vi "Substitute Actor.vi"(10 "Substitute Actor in":refnum<class "Actor.lvclass">, 11 "Current State Machine Actor":refnum<class "State Machine Actor.lvclass">) -> (0 "error out":errorcluster, 2 "Substitute Actor out":refnum<class "Actor.lvclass">)   [LabVIEW 2024]
doc: "(<B>Filename</B>: Actor Framework.lvlib:Actor.lvclass:Substitute Actor.vi)\n\nThis method copies information from the <b>Current Actor</b> to the <b>Substitute Actor</b>, including the to-self and the to-caller queue references. The purpose of this function is to allow an actor to define a method that replaces itself with another actor, useful for implementing a State Pattern Actor. Child classes should override this method to copy any additional fields that they need from the current to the substitute.\n\nThis method may return error code 678010: Illegal substitution. Overrides of this method may choose to return this error if the new actor is not one that is an appropriate substitute for the current actor, for whatever standards of \"appropriate\" are chosen for the current actor. If returning an error, override VIs should return the unmodified <b>Current Actor</b> as <b>Substitute Actor out</b>."
uses:
  State Machine Actor.lvclass/State Machine Actor.ctl
  State Machine Actor.lvclass
  C:/Users/uspoaotto/OneDrive - Oregon Tool/Desktop/working copies/stateMachineActor/src/_State Machine Actor/_State Machine Actor/_State Machine Actor.lvclass
  C:/Program Files (x86)/National Instruments/LabVIEW 2024/vi.lib/ActorFramework/Actor/Actor.lvclass
  C:/Users/uspoaotto/OneDrive - Oregon Tool/Desktop/working copies/stateMachineActor/src/State Machine Actor/State Machine Actor/State Machine Actor.lvclass
  <vilib>/ActorFramework/Actor/Actor.lvclass
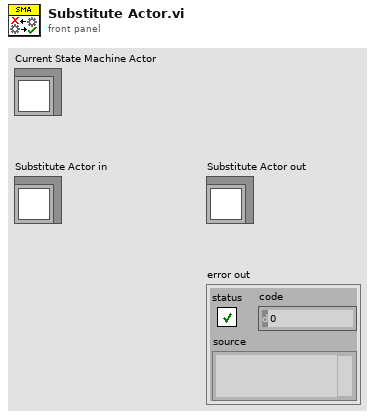
[diagram p1: front panel]
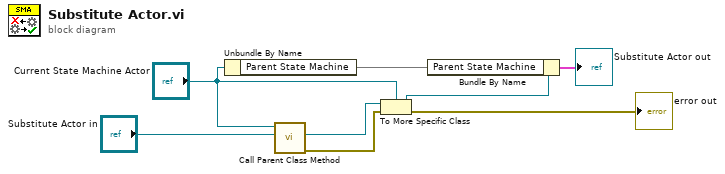
[diagram p0: block diagram]
diagram:
  n1 = Unbundle By Name("Current State Machine Actor") -> ("Parent State Machine"=w4)
  n2 = call-parent "Call Parent Class Method"("Substitute Actor in"="Substitute Actor in", "Current Actor"="Current State Machine Actor") -> ("error out"=w3:errorcluster, "Substitute Actor out"=w7:refnum<class "Actor.lvclass">)  [unwired: 8 in]
  n3 = To More Specific Class(target class="Current State Machine Actor", reference=w7, error in=w3) -> (specific class reference=w5:refnum<class "State Machine Actor.lvclass">, error out=→"error out":errorcluster)
  n4 = Bundle By Name(cluster=w5, "Parent State Machine"=w4) -> (→"Substitute Actor out":cluster{})
